vi "PS_Measure_Pol.vi"(7 "Number of Samples":i32=200, 8 "High Signal Extend":i32=50, 9 "Low Signal Start":i32=60, 10 "High Signal Start":i32=110, 11 "Sample Rate":dbl=1000.0) -> (0 "Data to Write":dbl, 1 "Optical Polarization":dbl format="%#.1f%", 2 "Corrected Low":dbl, 3 "Corrected High":dbl, 4 "Std Dev Low":dbl format="%.5f", 5 "Std Dev High":dbl format="%.5f")   [LabVIEW 2011]
uses:
  PS_Global.vi
  <vilib>/express/express shared/transition.llb/Dynamic To Waveform Array.vi
  <vilib>/express/express shared/transition.llb/Waveform Array To Dynamic.vi
  <vilib>/express/express arith-compare/Formula/Block/exnFormulaBlock how many pts in the wave.vi
  <vilib>/express/express shared/ex_Modify Signal Name.vi
  <vilib>/express/express arith-compare/Formula/XNode/ExpressFormulaBlockNode.xnode
panel:
  out "Data":dynamicdata(graph) caption="Section"
  out "Nuclear Polarization":dbl format="%#.1f%"
  out "Optical Polarization (%)":dynamicdata(graph)
  out "Mean Low":dbl format="%.4f"
  out "Mean High":dbl format="%.4f"
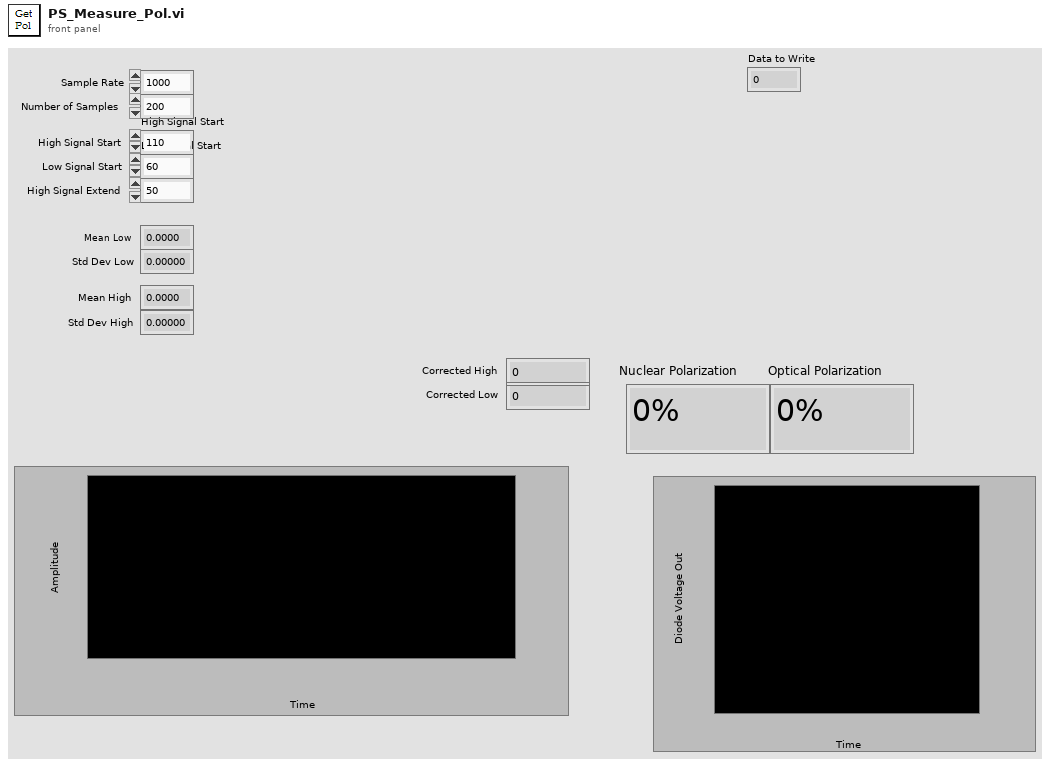
[diagram p1: front panel]
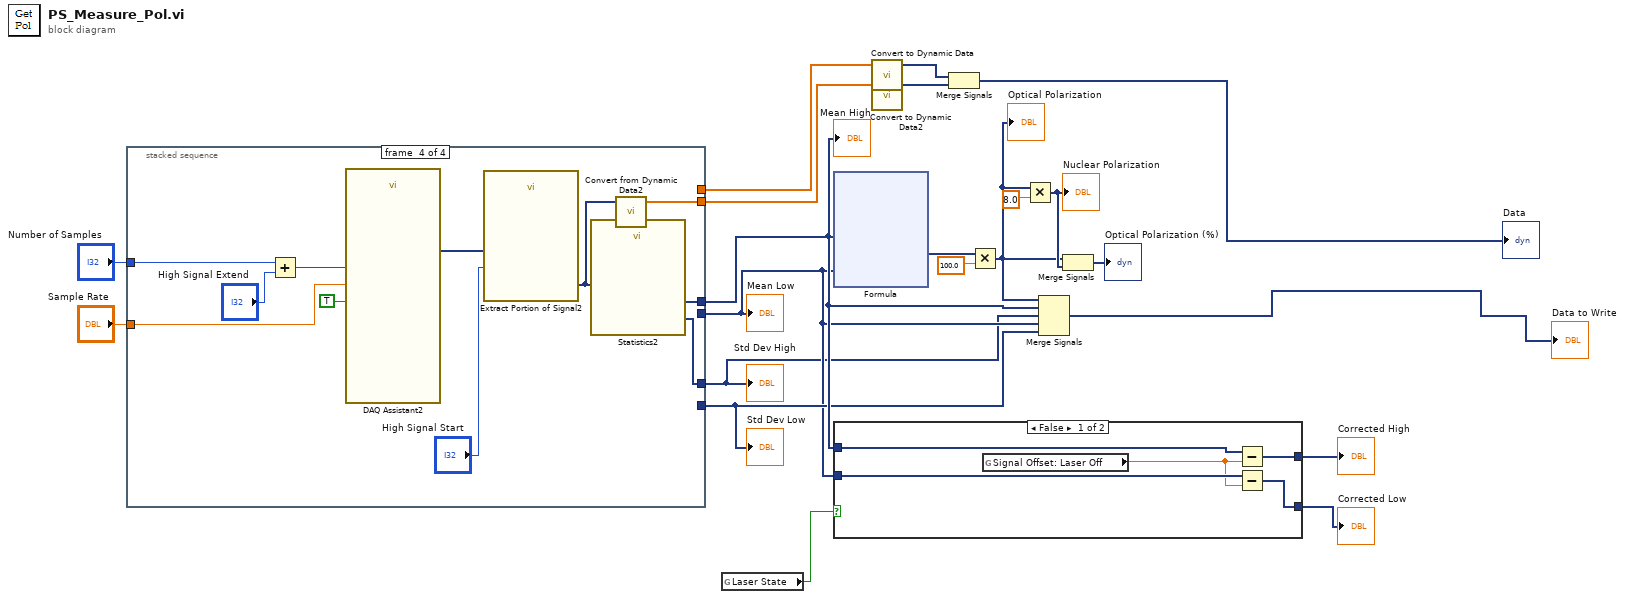
[diagram p0: block diagram]
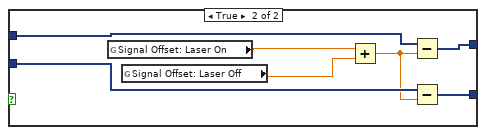
[diagram p2: hidden frame]
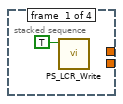
[diagram p3: hidden frame]
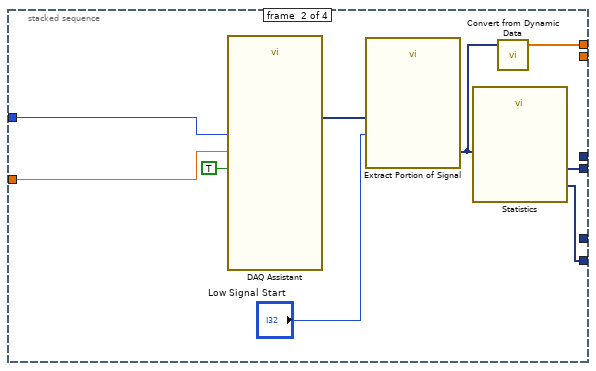
[diagram p4: hidden frame]
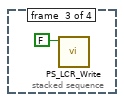
[diagram p5: hidden frame]
diagram:
  n1 = stacked-sequence {
    tunnel: [_ w26 _ _] -> w19
    tunnel: "Sample Rate" -> [_ w31 _ w43]
    tunnel: "Number of Samples" -> [_ w30 _ w35]
    tunnel: [_ _ _ w39] -> w18
    tunnel: [_ _ _ w37] -> w7
    tunnel: [_ w24 _ _] -> w5
    tunnel: [_ _ _ w36] -> w3
    tunnel: [_ w23 _ _] -> w6
    frame #0 {
      n2 = call "PS_LCR_Write.vi"("On/Off"=TRUE) -> ()  [unwired: 10 in, 1 out]
    }
    frame #1 {
      n3 = call "DAQ Assistant"("rate"=w31, "number of samples"=w30, "stop (F)"=TRUE) -> ("data"=w29:dynamicdata)  [unwired: 13 in, 3 out]
      n4 = call "Extract Portion of Signal"("Begin Sample"="Low Signal Start", "Signals"=w29) -> ("Section"=w25:dynamicdata)  [unwired: 8 in, 1 out]
      n5 = call "Statistics"("Signals"=w25) -> ("Standard Dev"=w23:dynamicdata, "Arithmetic Mean"=w24:dynamicdata)  [unwired: 24 in, 1 out]
      n6 = call "Convert from Dynamic Data"("Dynamic Data Type"=w25) -> ("Array"=w26:dbl[])  [unwired: 3 in]
    }
    frame #2 {
      n7 = call "PS_LCR_Write.vi"("On/Off"=FALSE) -> ()  [unwired: 10 in, 1 out]
    }
    frame #3 {
      n8 = Add(x=w35, y="High Signal Extend") -> (x+y=w33:i32)
      n9 = call "DAQ Assistant2"("rate"=w43, "number of samples"=w33, "stop (F)"=TRUE) -> ("data"=w42:dynamicdata)  [unwired: 13 in, 3 out]
      n10 = call "Extract Portion of Signal2"("Begin Sample"="High Signal Start", "Signals"=w42) -> ("Section"=w38:dynamicdata)  [unwired: 8 in, 1 out]
      n11 = call "Statistics2"("Signals"=w38) -> ("Standard Dev"=w36:dynamicdata, "Arithmetic Mean"=w37:dynamicdata)  [unwired: 24 in, 1 out]
      n12 = call "Convert from Dynamic Data2"("Dynamic Data Type"=w38) -> ("Array"=w39:dbl[])  [unwired: 3 in]
    }
  }
  "Mean High" <- w7
  "Mean Low" <- w5
  "Std Dev High" <- w3
  "Std Dev Low" <- w6
  n13 = global read "PS_Global.vi" "Laser State"() -> (w1:bool)
  n14 = xnode "Formula"("X1"=w7, "X2"=w5) -> ("Result"=w8:dynamicdata)  [unwired: 1 in, 1 out]
  n15 = case shown="False" w1 {
    tunnel: w5 -> [w46 w52]
    tunnel: w7 -> [w48 w53]
    tunnel: [w47 w55] -> w14
    tunnel: [w45 w54] -> w15
    frame False {
      n16 = global read "PS_Global.vi" "Signal Offset: Laser Off"() -> (w44:dbl)
      n17 = Subtract(x=w48, y=w44) -> (x-y=w47:dynamicdata)
      n18 = Subtract(x=w46, y=w44) -> (x-y=w45:dynamicdata)
    }
    frame True {
      n19 = global read "PS_Global.vi" "Signal Offset: Laser On"() -> (w50:dbl)
      n20 = global read "PS_Global.vi" "Signal Offset: Laser Off"() -> (w49:dbl)
      n21 = Add(x=w50, y=w49) -> (x+y=w51:dbl)
      n22 = Subtract(x=w53, y=w51) -> (x-y=w55:dynamicdata)
      n23 = Subtract(x=w52, y=w51) -> (x-y=w54:dynamicdata)
    }
  }
  "Corrected High" <- w14
  "Corrected Low" <- w15
  n24 = call "Convert to Dynamic Data"("Array"=w19) -> ("Dynamic Data Type"=w17:dynamicdata)  [unwired: 3 in]
  n25 = call "Convert to Dynamic Data2"("Array"=w18) -> ("Dynamic Data Type"=w16:dynamicdata)  [unwired: 3 in]
  n26 = Merge Signals(w17, w16) -> (→"Data":dynamicdata)
  n27 = Multiply(x=w8, y=100.0) -> (x*y=w11:dynamicdata)
  "Optical Polarization" <- w11
  n28 = Multiply(x=w11, y=8.0) -> (x*y=w13:dynamicdata)
  "Nuclear Polarization" <- w13
  n29 = Merge Signals(w11, w7, w3, w5, w6) -> (→"Data to Write":dynamicdata)
  n30 = Merge Signals(w11, w13) -> (→"Optical Polarization (%)":dynamicdata)
